vi "Script Add Constant VI --Library.vi"(4 "Project Ref":refnum<vi>, 6 "App Ref":refnum<vi>, 7 "Constant VI Name":string="TESTING.vi", 8 "error in":errorcluster, 9 "Constant VI Args":refnum<vi>, 10 "Library Reference":refnum<vi>) -> (0 "error out":errorcluster, 3 "Constant VI Path":path)   [LabVIEW 2020, in "ConstantErrorsMaker.lvlib"]
uses:
  ConstantErrorsMaker.lvlib
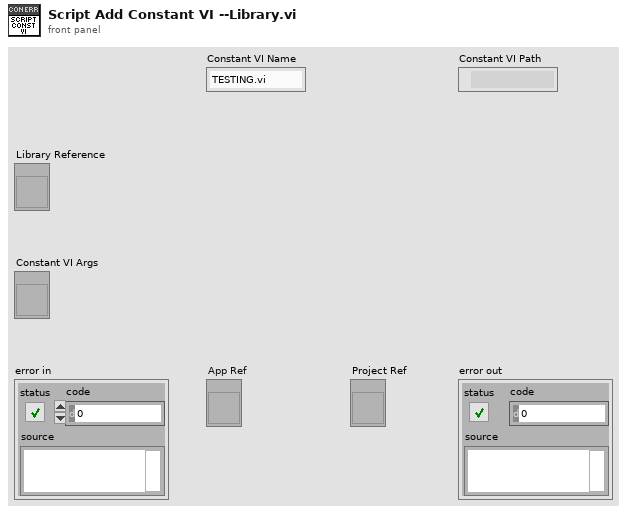
[diagram p1: front panel]
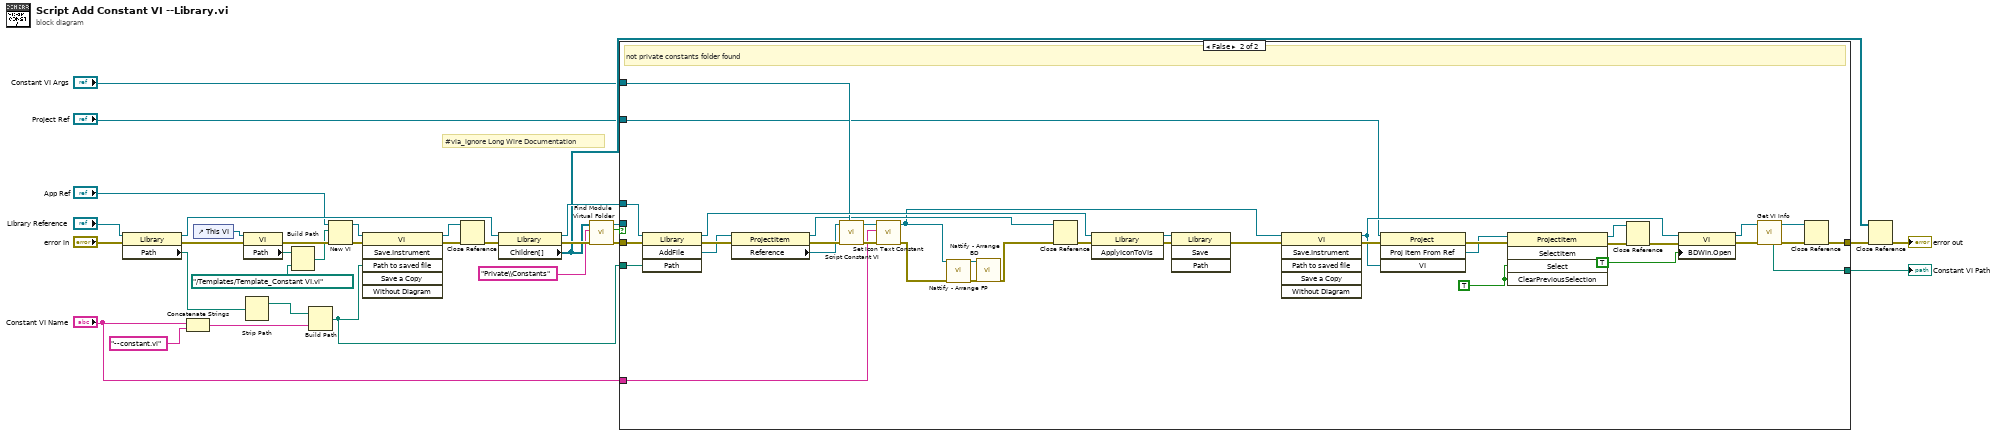
[diagram p0: block diagram]
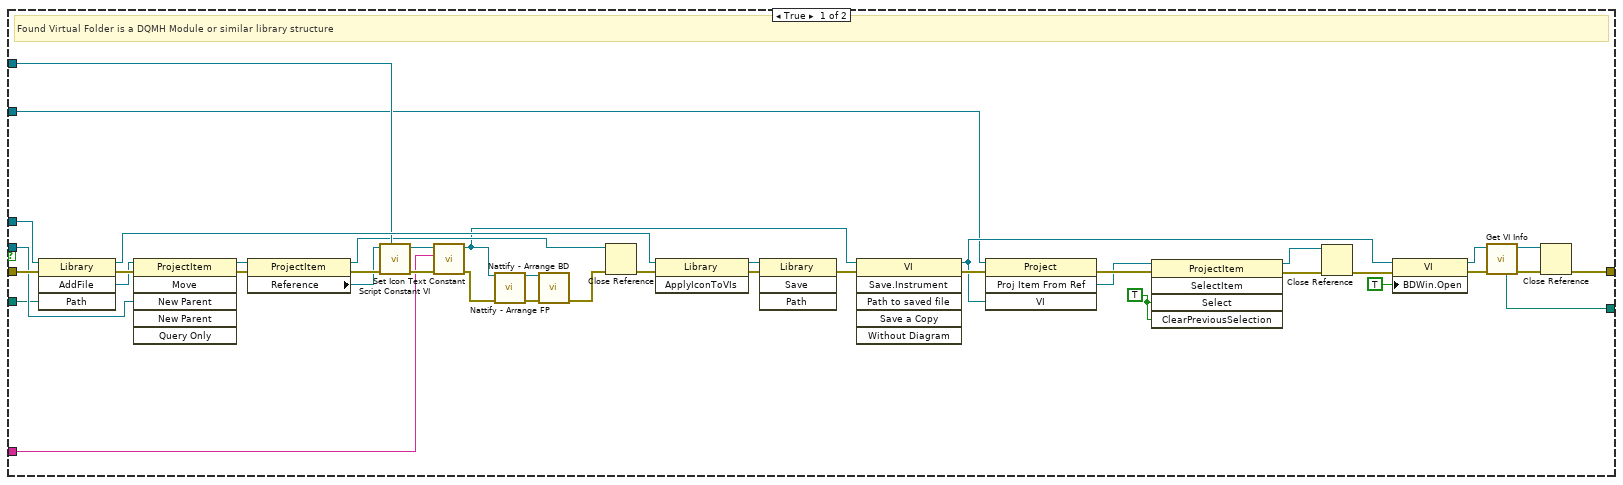
[diagram p2: hidden frame]
diagram:
  # "#via_ignore Long Wire Documentation"
  n1 = property class="Library"(reference="Library Reference", error in="error in") -> (reference out=w22:refnum<vi>, error out=w30:errorcluster, "Path"=w11:path)
  n2 = Concatenate Strings("Constant VI Name", "--constant.vi" ("input 1")) -> (w10:string)
  n3 = control-ref of="This VI"() -> (w9:refnum<vi>)
  n4 = property class="VI"(reference=w9, error in=w30) -> (error out=w24:errorcluster, "Path"=w8:path)  [unwired: 1 out]
  n5 = Strip Path(path=w11) -> (stripped path=w13:path)  [unwired: 1 out]
  n6 = Build Path(base path=w8, name or relative path=path "../Templates/Template_Constant VI.vi") -> (appended path=w7:path)
  n7 = Build Path(base path=w13, name or relative path=w10) -> (appended path=w12:path)
  n8 = New VI(8:w24, 10:w7, 11:"App Ref") -> (0:w27:errorcluster, 3:w15:refnum<vi>)  [unwired: 4 in]
  n9 = invoke class="VI" method="Save.Instrument"(reference=w15, error in=w27, "Path to saved file"=w12) -> (reference out=w5:refnum<vi>, error out=w25:errorcluster)  [unwired: 3 in, 4 out]
  n10 = Close Reference(reference=w5, error in (no error)=w25) -> (error out=w26:errorcluster)
  n11 = property class="Library"(reference=w22, error in=w26) -> (reference out=w23:refnum<vi>, error out=w32:errorcluster, "Children[]"=w19:refnum<vi>[])
  n12 = call "Find Module Virtual Folder.vi"("error in"=w32, "Virtual Folder"="Private\\Constants", "Children"=w19) -> ("error out"=w31:errorcluster, "Found?"=w20:bool, "ProjectItem out"=w21:refnum<vi>)  [unwired: 6 in]
  n13 = case shown="False" w20 {
    tunnel: [w63 w102] -> w33
    tunnel: w23 -> [w56 w95]
    tunnel: w31 -> [w74 w112]
    tunnel: w21 -> [w54 _]
    tunnel: "Constant VI Args" -> [w50 w90]
    tunnel: w12 -> [w51 w91]
    tunnel: "Constant VI Name" -> [w43 w84]
    tunnel: "Project Ref" -> [w38 w80]
    tunnel: [w34 w75] -> w2
    frame True {
      w41 = TRUE ("Select")
      # "Found Virtual Folder is a DQMH Module or similar library structure"
      n14 = invoke class="Library" method="AddFile"(reference=w56, error in=w74, "Path"=w51) -> (reference out=w53:refnum<vi>, error out=w73:errorcluster, "AddFile"=w55:refnum<vi>)  [unwired: 1 in, 1 out]
      n15 = invoke class="ProjectItem" method="Move"(reference=w55, error in=w73, "New Parent"=w54) -> (reference out=w48:refnum<vi>, error out=w70:errorcluster)  [unwired: 3 in, 4 out]
      n16 = property class="ProjectItem"(reference=w48, error in=w70) -> (reference out=w47:refnum<vi>, error out=w58:errorcluster, "Reference"=w37:refnum<vi>)
      n17 = call "Script Constant VI.vi"("Custom Argument Window"=w50, "error in"=w58, "VI Reference"=w37) -> ("error out"=w69:errorcluster, "VI reference"=w49:refnum<vi>)  [unwired: 7 in]
      n18 = call "Set Icon Text Constant.vi"("error in"=w69, "Text"=w43, "VI in"=w49) -> ("error out"=w67:errorcluster, "VI out"=w45:refnum<vi>)  [unwired: 7 in]
      n19 = call "Nattify - Arrange FP.vi"("VI in"=w45, "error in"=w67) -> ("VI out"=w46:refnum<vi>, "error out"=w68:errorcluster)  [unwired: 12 in]
      n20 = call "Nattify - Arrange BD.vi"("VI in"=w46, "error in"=w68) -> ("error out"=w65:errorcluster)  [unwired: 13 in]
      n21 = Close Reference(reference=w47, error in (no error)=w65) -> (error out=w71:errorcluster)
      n22 = invoke class="Library" method="ApplyIconToVIs"(reference=w53, error in=w71) -> (reference out=w52:refnum<vi>, error out=w72:errorcluster)  [unwired: 1 in, 1 out]
      n23 = invoke class="Library" method="Save"(reference=w52, error in=w72) -> (error out=w64:errorcluster)  [unwired: 2 in, 3 out]
      n24 = invoke class="VI" method="Save.Instrument"(reference=w45, error in=w64) -> (reference out=w40:refnum<vi>, error out=w61:errorcluster)  [unwired: 4 in, 4 out]
      n25 = invoke class="Project" method="Proj Item From Ref"(reference=w38, error in=w61, "VI"=w40) -> (error out=w62:errorcluster, "ProjItemFromRef"=w42:refnum<vi>)  [unwired: 1 in, 2 out]
      n26 = invoke class="ProjectItem" method="SelectItem"(reference=w42, error in=w62, "Select"=w41, "ClearPreviousSelection"=w41) -> (reference out=w39:refnum<vi>, error out=w60:errorcluster)  [unwired: 1 in, 3 out]
      n27 = Close Reference(reference=w39, error in (no error)=w60) -> (error out=w59:errorcluster)
      n28 = property class="VI"(reference=w40, error in=w59, "BDWin.Open"=TRUE ("Block Diagram Window:Open")) -> (reference out=w36:refnum<vi>, error out=w66:errorcluster)
      n29 = call "Get VI Info.vi"("error in"=w66, "VI in"=w36) -> ("error out"=w57:errorcluster, "VI out"=w35:refnum<vi>, "VI Path"=w34:path)  [unwired: 4 in, 3 out]
      n30 = Close Reference(reference=w35, error in (no error)=w57) -> (error out=w63:errorcluster)
    }
    frame False {
      w82 = TRUE ("Select")
      # "not private constants folder found"
      n31 = invoke class="Library" method="AddFile"(reference=w95, error in=w112, "Path"=w91) -> (reference out=w93:refnum<vi>, error out=w101:errorcluster, "AddFile"=w94:refnum<vi>)  [unwired: 1 in, 1 out]
      n32 = property class="ProjectItem"(reference=w94, error in=w101) -> (reference out=w88:refnum<vi>, error out=w108:errorcluster, "Reference"=w78:refnum<vi>)
      n33 = call "Script Constant VI.vi"("Custom Argument Window"=w90, "error in"=w108, "VI Reference"=w78) -> ("error out"=w109:errorcluster, "VI reference"=w89:refnum<vi>)  [unwired: 7 in]
      n34 = call "Set Icon Text Constant.vi"("error in"=w109, "Text"=w84, "VI in"=w89) -> ("error out"=w106:errorcluster, "VI out"=w86:refnum<vi>)  [unwired: 7 in]
      n35 = call "Nattify - Arrange FP.vi"("VI in"=w86, "error in"=w106) -> ("VI out"=w87:refnum<vi>, "error out"=w107:errorcluster)  [unwired: 12 in]
      n36 = call "Nattify - Arrange BD.vi"("VI in"=w87, "error in"=w107) -> ("error out"=w104:errorcluster)  [unwired: 13 in]
      n37 = Close Reference(reference=w88, error in (no error)=w104) -> (error out=w110:errorcluster)
      n38 = invoke class="Library" method="ApplyIconToVIs"(reference=w93, error in=w110) -> (reference out=w92:refnum<vi>, error out=w111:errorcluster)  [unwired: 1 in, 1 out]
      n39 = invoke class="Library" method="Save"(reference=w92, error in=w111) -> (error out=w103:errorcluster)  [unwired: 2 in, 3 out]
      n40 = invoke class="VI" method="Save.Instrument"(reference=w86, error in=w103) -> (reference out=w81:refnum<vi>, error out=w99:errorcluster)  [unwired: 4 in, 4 out]
      n41 = invoke class="Project" method="Proj Item From Ref"(reference=w80, error in=w99, "VI"=w81) -> (error out=w100:errorcluster, "ProjItemFromRef"=w83:refnum<vi>)  [unwired: 1 in, 2 out]
      n42 = invoke class="ProjectItem" method="SelectItem"(reference=w83, error in=w100, "Select"=w82, "ClearPreviousSelection"=w82) -> (reference out=w79:refnum<vi>, error out=w98:errorcluster)  [unwired: 1 in, 3 out]
      n43 = Close Reference(reference=w79, error in (no error)=w98) -> (error out=w97:errorcluster)
      n44 = property class="VI"(reference=w81, error in=w97, "BDWin.Open"=TRUE ("Block Diagram Window:Open")) -> (reference out=w77:refnum<vi>, error out=w105:errorcluster)
      n45 = call "Get VI Info.vi"("error in"=w105, "VI in"=w77) -> ("error out"=w96:errorcluster, "VI out"=w76:refnum<vi>, "VI Path"=w75:path)  [unwired: 4 in, 3 out]
      n46 = Close Reference(reference=w76, error in (no error)=w96) -> (error out=w102:errorcluster)
    }
  }
  "Constant VI Path" <- w2
  n47 = Close Reference(reference=w19, error in (no error)=w33) -> (error out=→"error out":errorcluster)
